vi "Init.vi"(8 "error in (no error)":errorcluster, 10 "Channel":i16, 11 "TrialBasedExperiment in":refnum<class "OriDiscExperiment.lvclass">) -> (0 "error out":errorcluster, 3 "TrialBasedExperiment out":refnum<class "OriDiscExperiment.lvclass">)   [LabVIEW 2014, in "OriDiscExperiment.lvclass"]
uses:
  OriDiscExperiment.lvclass
  StartTrial.vi
  TwoAfcEye/TwoAfcEye.lvclass
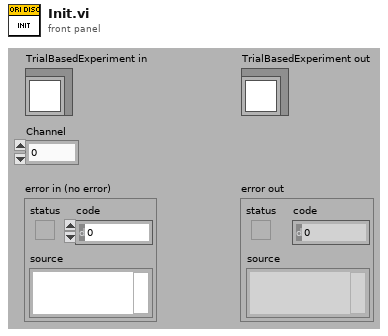
[diagram p1: front panel]
types:
  T1 = cluster{"Intertrial":dbl, "AcquireFixation":dbl, "HoldFixation":dbl, "DelayPeriod":dbl, "ResponsePeriod":dbl}
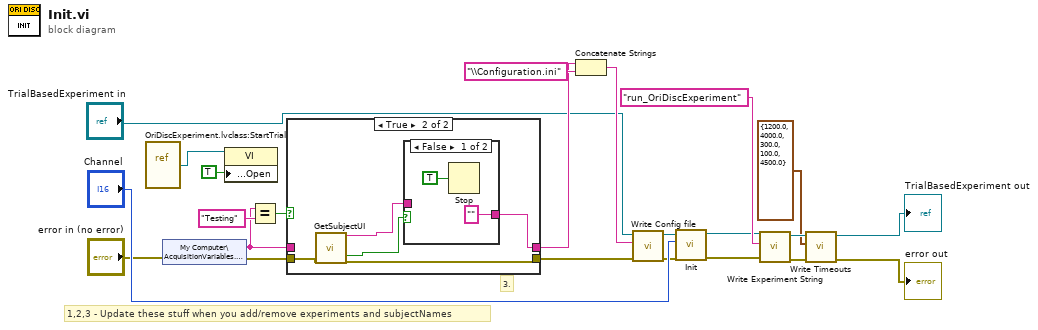
[diagram p0: block diagram]
diagram:
  # "1,2,3 - Update these stuff when you add/remove experiments and subjectNames"
  # "3."
  n1 = vi-ref "OriDiscExperiment.lvclass:StartTrial.vi"() -> (w2:refnum<vi>)
  n2 = shared-variable "My Computer\\AcquisitionVariables.lvlib\\Subject"(error in="error in (no error)") -> (w19:string, error out=w18:errorcluster)
  n3 = property class="VI"(reference=w2, "Front Panel.Open"=TRUE ("Front Panel Window:Open")) -> ()  [unwired: 1 in, 2 out]
  n4 = Equal?(x=w19, y="Testing") -> (x = y?=w21:bool)
  n5 = case shown="True" w21 {
    tunnel: [w25 w30] -> w16
    tunnel: w19 -> [w25 _]
    tunnel: w18 -> [w24 w26]
    tunnel: [w24 w27] -> w17
    frame False {
    }
    frame True {
      n6 = call "GetSubjectUI.vi"("error in (no error)"=w26) -> ("subjectSelected"=w29:string, "OK"=w28:bool, "error out"=w27:errorcluster)  [unwired: 16 in]
      n7 = case shown="False" w28 {
        tunnel: w29 -> [_ w33]
        tunnel: ["" ("subjectSelected") w33] -> w30
        frame False {
          n8 = Stop(stop? (T)=TRUE) -> ()
        }
        frame True {
        }
      }
    }
  }
  n9 = Concatenate Strings(w16, "\\Configuration.ini") -> (w23:string)
  n10 = call-dynamic "Write Config file.vi"("error in (no error)"=w17, "Config file"=w23, "TrialBasedExperiment in"="TrialBasedExperiment in") -> ("error out"=w12:errorcluster, "TrialBasedExperiment out"=w13:refnum<class "OriDiscExperiment.lvclass">)  [unwired: 7 in]
  n11 = call-parent "Init.vi"("error in (no error)"=w12, "Channel"="Channel", "TrialBasedExperiment in"=w13) -> ("error out"=w6:errorcluster, "TrialBasedExperiment out"=w7:refnum<class "OriDiscExperiment.lvclass">)  [unwired: 7 in]
  n12 = call-dynamic "Write Experiment String.vi"("error in (no error)"=w6, "Experiment String"="run_OriDiscExperiment" ("string"), "TrialBasedExperiment in"=w7) -> ("error out"=w10:errorcluster, "TrialBasedExperiment out"=w11:refnum<class "OriDiscExperiment.lvclass">)  [unwired: 7 in]
  n13 = call-dynamic "Write Timeouts.vi"("error in (no error)"=w10, "Timeouts"=T1 {"Intertrial"=1200.0, "AcquireFixation"=4000.0, "HoldFixation"=300.0, "DelayPeriod"=100.0, "ResponsePeriod"=4500.0}, "TrialBasedExperiment in"=w11) -> ("error out"=→"error out":errorcluster, "TrialBasedExperiment out"=→"TrialBasedExperiment out":refnum<class "OriDiscExperiment.lvclass">)  [unwired: 7 in]
